vi "Example - Building a DLL.vi"() -> ()   [LabVIEW 2020]
doc: "Demonstrates the use of the Application Builder API to create and build a Shared Library build specification."
uses:
  <vilib>/AppBuilder/AB_API/common/AB_API Version Number.ctl
  <vilib>/AppBuilder/AB_API/DLL/NI_AB_API_DLL.lvclass
panel:
  out "Generated Files":path[](array[path])
  # "Overview: Demonstrates the use of the Application Builder API to create and build a Shared Library build specification.\nRequirements: LabVIEW Professional Development System or LabVIEW Application Builder\nInstructions:\n1. Run the VI. A Shared Library (DLL) build specification will be created, which will then be built programmatically.\n2. Examine the DLL build specification in the new project.\n3. Close the temporary project and delete the temporary project files generated by this example when you are done."
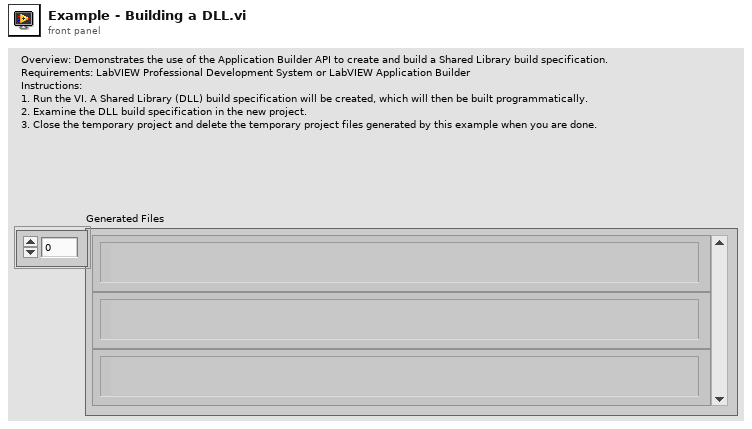
[diagram p1: front panel]
types:
  T1 = typedef "AB_API Version Number.ctl" = cluster{"Major":u16, "Minor":u16, "Fix":u16, "Build":u16}
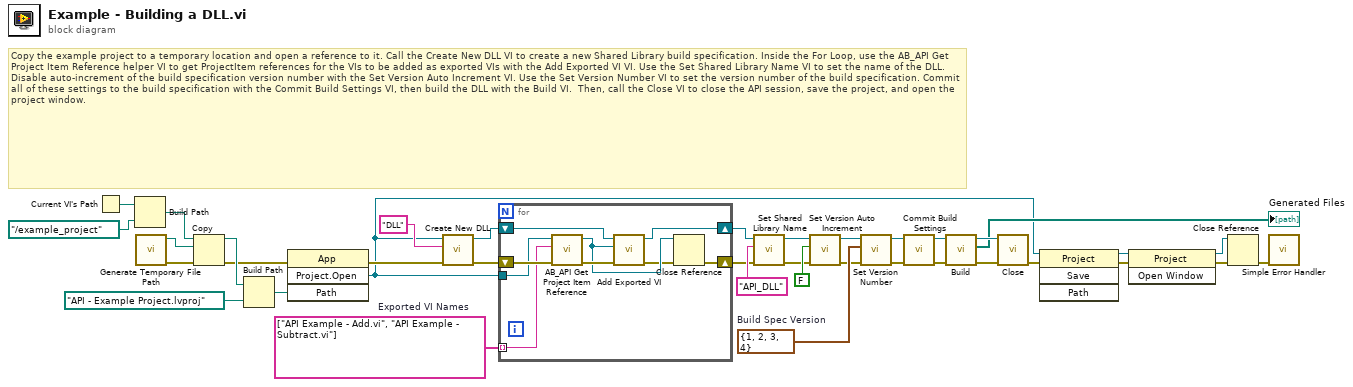
[diagram p0: block diagram]
diagram:
  w11 = T1 {"Major"=1, "Minor"=2, "Fix"=3, "Build"=4}  # Build Spec Version
  w25 = string[] ["API Example - Add.vi", "API Example - Subtract.vi"]  # Exported VI Names
  # "Copy the example project to a temporary location and open a reference to it. Call the Create New DLL VI to create a new Shared Library build specification. Inside the For Loop, use the AB_API Get Project Item Reference helper VI to get ProjectItem references for the VIs to be added as exported VIs with the Add Exported VI VI. Use the Set Shared Library Name VI to set the name of the DLL. Disable auto-increment of the build specification version number with the Set Version Auto Increment VI. Use the Set Version Number VI to set the version number of the build specification. Commit all of these settings to the build specification with the Commit Build Settings VI, then build the DLL with the Build VI.  Then, call the Close VI to close the API session, save the project, and open the project window."
  n1 = Current VI's Path() -> (path=w24:path)
  n2 = Build Path(base path=w24, name or relative path=path "../example_project" ("path")) -> (appended path=w20:path)
  n3 = call <vilib>:"Generate Temporary File Path.vi"() -> ("error out"=w13:errorcluster, "Unique Temporary File Path"=w19:path)  [unwired: 10 in]
  n4 = Copy(8:w13, 10:w19, 11:w20) -> (0:w12:errorcluster, 3:w18:path)  [unwired: 2 in, 1 out]
  n5 = Build Path(base path=w18, name or relative path=path "API - Example Project.lvproj") -> (appended path=w16:path)
  n6 = invoke class="App" method="Project.Open"(error in=w12, "Path"=w16) -> (error out=w23:errorcluster, "Project:Open"=w15:refnum<vi>)  [unwired: 2 in, 2 out]
  n7 = call <vilib>:"Create New DLL.vi"("error in (no error)"=w23, "Build specification name"="DLL", "Project Refnum"=w15) -> ("error out"=w36:errorcluster, "DLL out"=w37:refnum<class "NI_AB_API_DLL.lvclass">)  [unwired: 7 in]
  n8 = for {
    shift-right: [w45] -> w29
    shift-left: w37 -> [w38]
    shift-right: [w46] -> w30
    shift-left: w36 -> [w44]
    tunnel: w15 -> [w41]
    tunnel: w25 -> [w40] mode=indexing
    n9 = call <vilib>:"AB_API Get Project Item Reference.vi"("error in (no error)"=w44, "Name"=w40, "Project Refnum"=w41) -> ("error out"=w43:errorcluster, "ProjectItem Refnum"=w42:refnum<vi>)  [unwired: 6 in, 1 out]
    n10 = call-dynamic "Add Exported VI.vi"("error in (no error)"=w43, "ProjectItem Refnum"=w42, "DLL in"=w38) -> ("error out"=w39:errorcluster, "DLL out"=w45:refnum<class "NI_AB_API_DLL.lvclass">)  [unwired: 7 in]
    n11 = Close Reference(reference=w42, error in (no error)=w39) -> (error out=w46:errorcluster)
  }
  n12 = call-dynamic "Set Shared Library Name.vi"("error in (no error)"=w30, "Shared library file name"="API_DLL" ("Name"), "DLL in"=w29) -> ("error out"=w7:errorcluster, "DLL out"=w4:refnum<class "NI_AB_API_DLL.lvclass">)  [unwired: 7 in]
  n13 = call-dynamic "Set Version Auto Increment.vi"("error in (no error)"=w7, "Auto Increment Version"=FALSE, "NI_AB_API_DLL in"=w4) -> ("error out"=w10:errorcluster, "NI_AB_API_DLL out"=w9:refnum<class "NI_AB_API_DLL.lvclass">)  [unwired: 7 in]
  n14 = call-dynamic "Set Version Number.vi"("error in (no error)"=w10, "Version number"=w11, "DLL in"=w9) -> ("error out"=w6:errorcluster, "DLL out"=w5:refnum<class "NI_AB_API_DLL.lvclass">)  [unwired: 7 in]
  n15 = call-dynamic "Commit Build Settings.vi"("error in (no error)"=w6, "DLL in"=w5) -> ("error out"=w35:errorcluster, "DLL out"=w34:refnum<class "NI_AB_API_DLL.lvclass">)  [unwired: 8 in]
  n16 = call-dynamic "Build.vi"("error in (no error)"=w35, "DLL in"=w34) -> ("error out"=w32:errorcluster, "GeneratedFiles"=→"Generated Files":path[], "DLL out"=w33:refnum<class "NI_AB_API_DLL.lvclass">)  [unwired: 6 in, 1 out]
  n17 = call-dynamic "Close.vi"("error in (no error)"=w32, "DLL in"=w33) -> ("error out"=w27:errorcluster)  [unwired: 9 in]
  n18 = invoke class="Project" method="Save"(reference=w15, error in=w27) -> (reference out=w2:refnum<vi>, error out=w28:errorcluster)  [unwired: 2 in, 2 out]
  n19 = invoke class="Project" method="Open Window"(reference=w2, error in=w28) -> (reference out=w1:refnum<vi>, error out=w3:errorcluster)  [unwired: 1 in, 1 out]
  n20 = Close Reference(reference=w1, error in (no error)=w3) -> (error out=w22:errorcluster)
  n21 = call <vilib>:"Simple Error Handler.vi"("error in (no error)"=w22) -> ()  [unwired: 4 in, 5 out]
